vi "GetCursorPos.vi"(8 "error in":errorcluster) -> (0 "error out":errorcluster, 11 "Position":cluster{"X":i32, "Y":i32})   [LabVIEW 2020]
uses:
  user32.dll
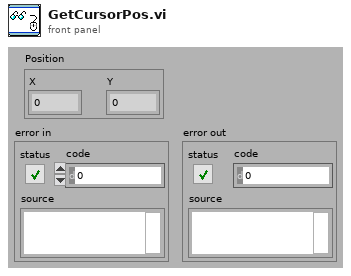
[diagram p1: front panel]
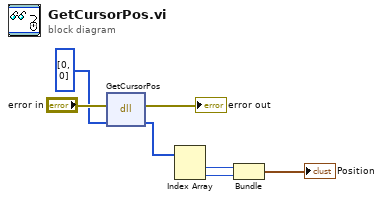
[diagram p0: block diagram]
diagram:
  n1 = dll-call lib="user32.dll" fn="GetCursorPos"(error in="error in", "POINT"=i32[] [0, 0] ("dx")) -> (error out=→"error out":errorcluster, "POINT"=w4:i32[])  [unwired: 3 in, 1 out]
  n2 = Index Array(array=w4) -> (element #1=w3:i32, element #2=w2:i32)  [unwired: 2 in]
  n3 = Bundle(w3, w2) -> (→"Position":cluster{i32, i32})  [unwired: 1 in]
